vi "Read Retry on Timeout.vi"(11 "CIF_DAQ_DVR_Multi in":refnum<class "CIF_DAQ_DVR_Multi.lvclass">) -> (2 "FIFO Retry on Timeout":bool, 3 "CIF_DAQ_DVR_Multi out":refnum<class "CIF_DAQ_DVR_Multi.lvclass">)   [LabVIEW 2021, in "CIF_DAQ_DVR_Multi.lvclass"]
uses:
  CIF_DAQ_DVR_Multi.lvclass
  CIF_DAQ_DVR_Multi.lvclass/CIF_DAQ_DVR_Multi.ctl
  FIFO_DAQ_DVR/CIF_NIChn_FIFO_DAQ_DVR.lvclass
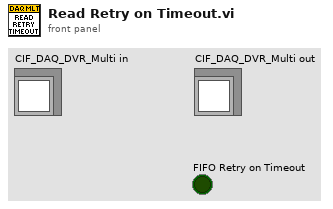
[diagram p1: front panel]
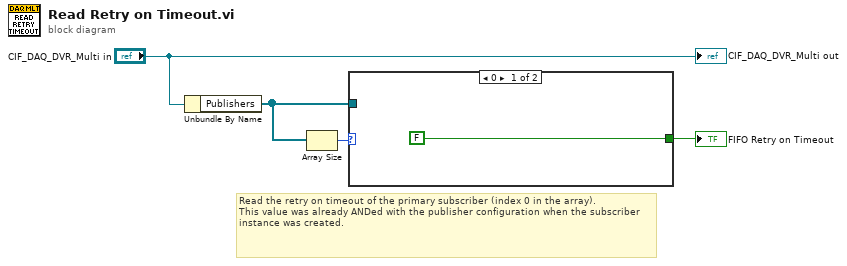
[diagram p0: block diagram]
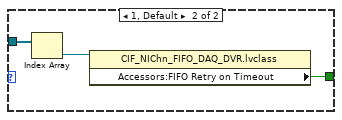
[diagram p2: hidden frame]
diagram:
  # "Read the retry on timeout of the primary subscriber (index 0 in the array).  \nThis value was already ANDed with the publisher configuration when the subscriber instance was created."
  n1 = Unbundle By Name("CIF_DAQ_DVR_Multi in") -> ("Publishers"=w2:refnum<class "CIF_NIChn_FIFO_DAQ_DVR.lvclass">[])
  n2 = Array Size(array=w2) -> (size(s)=w1:i32)
  n3 = case shown="0" w1 {
    tunnel: [FALSE ("Accessors:FIFO Retry on Timeout") w8] -> w3
    tunnel: w2 -> [_ w6]
    frame 0 {
    }
    frame 1, Default {
      n4 = Index Array(array=w6) -> (element=w7:refnum<class "CIF_NIChn_FIFO_DAQ_DVR.lvclass">)  [unwired: 1 in]
      n5 = property class="CIF_NIChn_FIFO_DAQ_DVR.lvclass"(reference=w7) -> ("Accessors:FIFO Retry on Timeout"=w8:bool)  [unwired: 1 in, 2 out]
    }
  }
  "FIFO Retry on Timeout" <- w3
  "CIF_DAQ_DVR_Multi out" <- "CIF_DAQ_DVR_Multi in"
